vi "测试文件.vi"() -> ()   [LabVIEW 2017]
panel:
  out "deleted portion":dbl[](array[numeric])
  out "array w/ subset deleted":dbl[](array[numeric])
  in  "Array":dbl[](array[numeric])
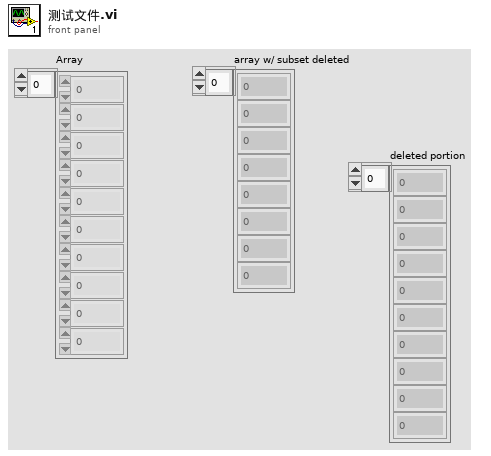
[diagram p1: front panel]
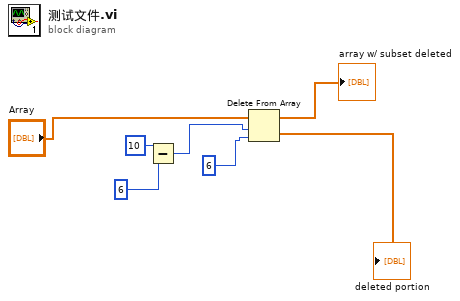
[diagram p0: block diagram]
diagram:
  n1 = Subtract(x=10, y=6) -> (x-y=w3:i32)
  n2 = Delete From Array(array="Array", length=w3, index=6) -> (deleted portion=→"deleted portion":dbl[], array with subset deleted=→"array w/ subset deleted":dbl[])
